vi "nominal dataset list.vi"(8 "error in (no error)":errorcluster, 9 "out_count":u32, 10 "out_list":i32, 11 "client":i32) -> (0 "error out":errorcluster, 1 "out_count out":u32, 2 "out_list out":i32, 3 "function return":i32)   [LabVIEW 2020, in "client.lvlib"]
doc: "int32_t nominal_dataset_list(int32_t client, int32_t *out_list, uint32_t *out_count);"
uses:
  client.lvlib
  bin/nominalClient_64.dll
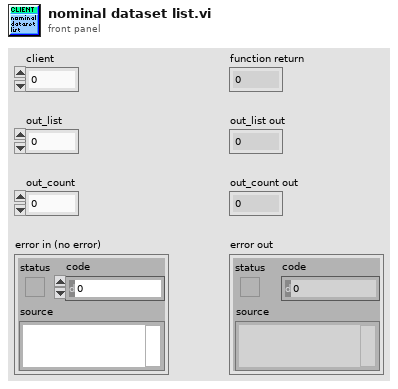
[diagram p1: front panel]
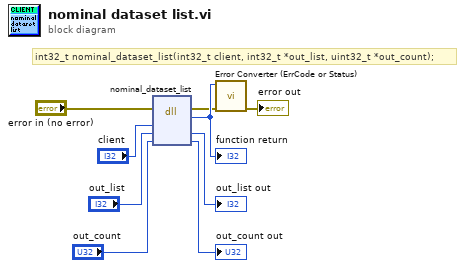
[diagram p0: block diagram]
diagram:
  # "int32_t nominal_dataset_list(int32_t client, int32_t *out_list, uint32_t *out_count);"
  n1 = dll-call lib="C:/code/labview-client-rs/lv_src/bin/nominalClient_*.*" fn="nominal_dataset_list"(error in="error in (no error)", "client"="client", "out_list"="out_list", "out_count"="out_count") -> (error out=w2:errorcluster, w9:i32, "out_list"=→"out_list out":i32, "out_count"=→"out_count out":u32)  [unwired: 3 in, 1 out]
  "function return" <- w9
  n2 = call "Error Converter (ErrCode or Status).vi"("error in (no error)"=w2, "error code"=w9) -> ("error out"=→"error out":errorcluster)  [unwired: 9 in]
